vi "in_spline y1 to coefficients.vi"(9 "Y1":dbl[](array[numeric]), 10 "X":dbl[](array[numeric]), 11 "Y":dbl[](array[numeric])) -> (3 "coefficients":dbl[][](array[numeric]))   [LabVIEW 2010, in "NI_Gmath.lvlib"]
uses:
  NI_Gmath.lvlib
  in_diff and divided diff (dx).vi
  in_diff and divided diff (dy over dx).vi
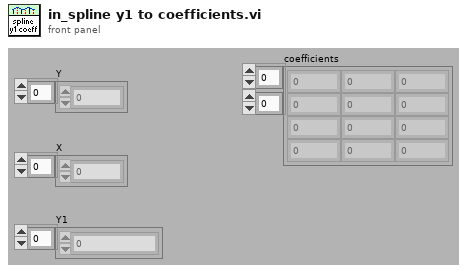
[diagram p1: front panel]
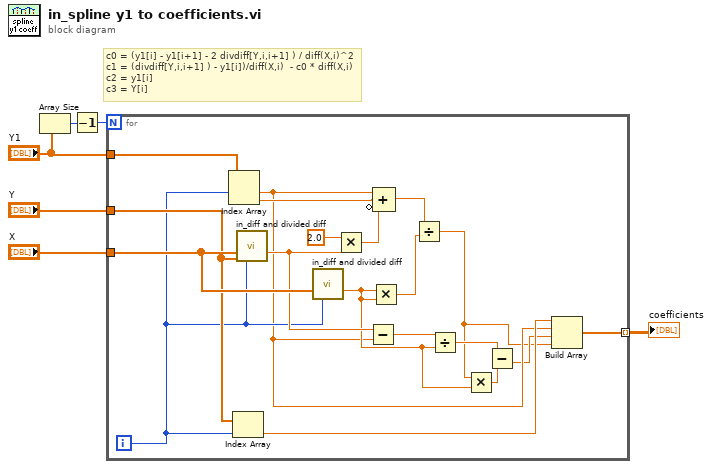
[diagram p0: block diagram]
diagram:
  # "c0 = (y1[i] - y1[i+1] - 2 divdiff[Y,i,i+1] ) / diff(X,i)^2\nc1 = (divdiff[Y,i,i+1] ) - y1[i])/diff(X,i)  - c0 * diff(X,i)\nc2 = y1[i]\nc3 = Y[i]"
  n1 = Array Size(array="Y1") -> (size(s)=w4:i32)
  n2 = Decrement(x=w4) -> (x-1=w3:i32)
  n3 = for {
    N: w3 -> [_]
    tunnel: "Y" -> [w13]
    tunnel: "X" -> [w21]
    tunnel: "Y1" -> [w25]
    tunnel: [w12] -> w1 mode=indexing
    i -> [w11]
    n4 = Index Array(array=w25, index #1=w11) -> (element #1=w9:dbl, element #2=w24:dbl)  [unwired: 1 in]
    n5 = Index Array(array=w13, index=w11) -> (element=w10:dbl)
    n6 = call-poly "in_diff and divided diff.vi"("X"=w21, "Y"=w13, "i1"=w11) -> ("difference"=w18:dbl)  [unwired: 12 in]
    n7 = call-poly "in_diff and divided diff.vi"("X"=w21, "i1"=w11) -> ("difference"=w15:dbl)  [unwired: 13 in]
    n8 = Multiply(x=2.0, y=w18) -> (x*y=w22:dbl)
    n9 = Subtract(x=w18, y=w9) -> (x-y=w17:dbl)
    n10 = Multiply(x=w15, y=w15) -> (x*y=w19:dbl)
    n11 = Compound Arithmetic op=ADD(w9, w24, invert w22) -> (w20:dbl)
    n12 = Divide(x=w20, y=w19) -> (x/y=w7:dbl)
    n13 = Divide(x=w17, y=w15) -> (x/y=w16:dbl)
    n14 = Multiply(x=w7, y=w15) -> (x*y=w14:dbl)
    n15 = Subtract(x=w16, y=w14) -> (x-y=w8:dbl)
    n16 = Build Array(w10, w9, w8, w7) -> (w12:dbl[])
  }
  "coefficients" <- w1
